vi "api_SetString.vi"(7 "group":string, 8 "error in (no error)":errorcluster, 9 "string_in":string, 10 "param":string, 11 "ConfigClass_DVR":refnum<data-value>) -> (0 "error out":errorcluster, 3 "ConfigClass_DVR_out":refnum<data-value>)   [LabVIEW 2019, in "ConfigClass.lvlib" / "ConfigClass.lvclass"]
uses:
  ConfigClass.lvclass
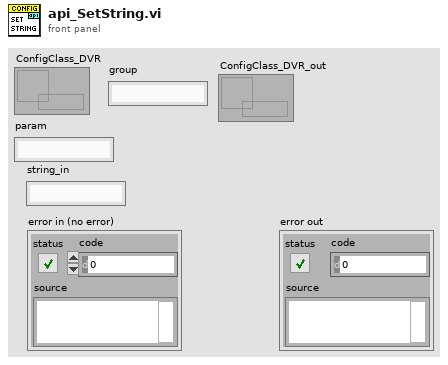
[diagram p1: front panel]
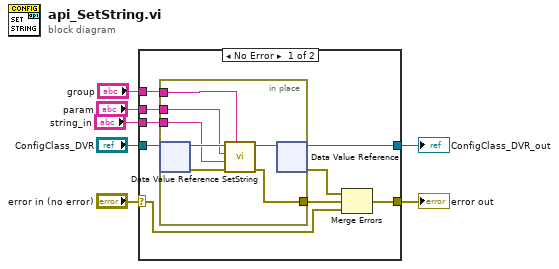
[diagram p0: block diagram]
diagram:
  n1 = case shown="No Error" "error in (no error)" {
    selector: "error in (no error)" -> [w10 w25]
    tunnel: "ConfigClass_DVR" -> [w16 w24]
    tunnel: [w13 w25] -> w6
    tunnel: [w12 w24] -> w4
    tunnel: "param" -> [w11 _]
    tunnel: "string_in" -> [w9 _]
    tunnel: "group" -> [w8 _]
    frame No Error {
      n2 = in-place {
        in-place-border: [w21] -> w14
        in-place-border: w11 -> [w19]
        in-place-border: w9 -> [w18]
        in-place-border: w8 -> [w17]
        n3 = in-place-dvr #1(w16) -> (w23:refnum<class "ConfigClass.lvclass">, w20:errorcluster)
        n4 = call-dynamic "SetString.vi"("group"=w17, "error in (no error)"=w20, "string_in"=w18, "param"=w19, "ConfigClass_IN"=w23) -> ("error out"=w21:errorcluster, "ConfigClass_OUT"=w22:refnum<class "ConfigClass.lvclass">)  [unwired: 5 in]
        n5 = in-place-dvr #1(w22) -> (w12:refnum<data-value>, w15:errorcluster)
      }
      n6 = Merge Errors(w15, w14, w10) -> (w13:errorcluster)
    }
    frame Error {
    }
  }
  "ConfigClass_DVR_out" <- w4
  "error out" <- w6
